vi "Inverter_write_read_json text step array.vi"(8 "error in":errorcluster, 9 "json_array_from_file":T1[](array[typedef])=[{"step_description (prompt)"="(prompt)", "save results"=FALSE, "step_type"=enum."prompt", "Step_name"="", "bool"=[], "data_unit"=enum."bool", "dbl"=[], "I32"=[], "string"=[]}, {"step_description (prompt)"="set hipot Voltage", "save results"=FALSE, "step_type"=enum."wait (sec)", "Step_name"="", "bool"=[], "data_unit"=enum."DBL", "dbl"=[], "I32"=[], "string"=[]}, {"step_description (prompt)"="read hipot v", "save results"=FALSE, "step_type"=enum."default", "Step_name"="", "bool"=[], "data_unit"=enum."bool", "dbl"=[], "I32"=[], "string"=[]}] {"dbl" format="%.3f"}, 10 "write_read":T4=enum."read", 11 "File Path":path) -> (0 "error out":errorcluster, 1 "steps array out":T1[](array[typedef]) {"dbl" format="%.3f"}, 3 "File Path":path)   [LabVIEW 2020]
uses:
  controls/Inverter_step.ctl
  controls/Inverter_step_type.ctl
  MPB/controls/data type.ctl
  MPB/controls/write_read.ctl
  3e47bdee-b09f-426d-96e8-78c270cf6aec.vi
  <vilib>/JDP Science/JSONtext/JSON text to Variant.vi
  <vilib>/JDP Science/JSONtext/JSONtext.lvlib
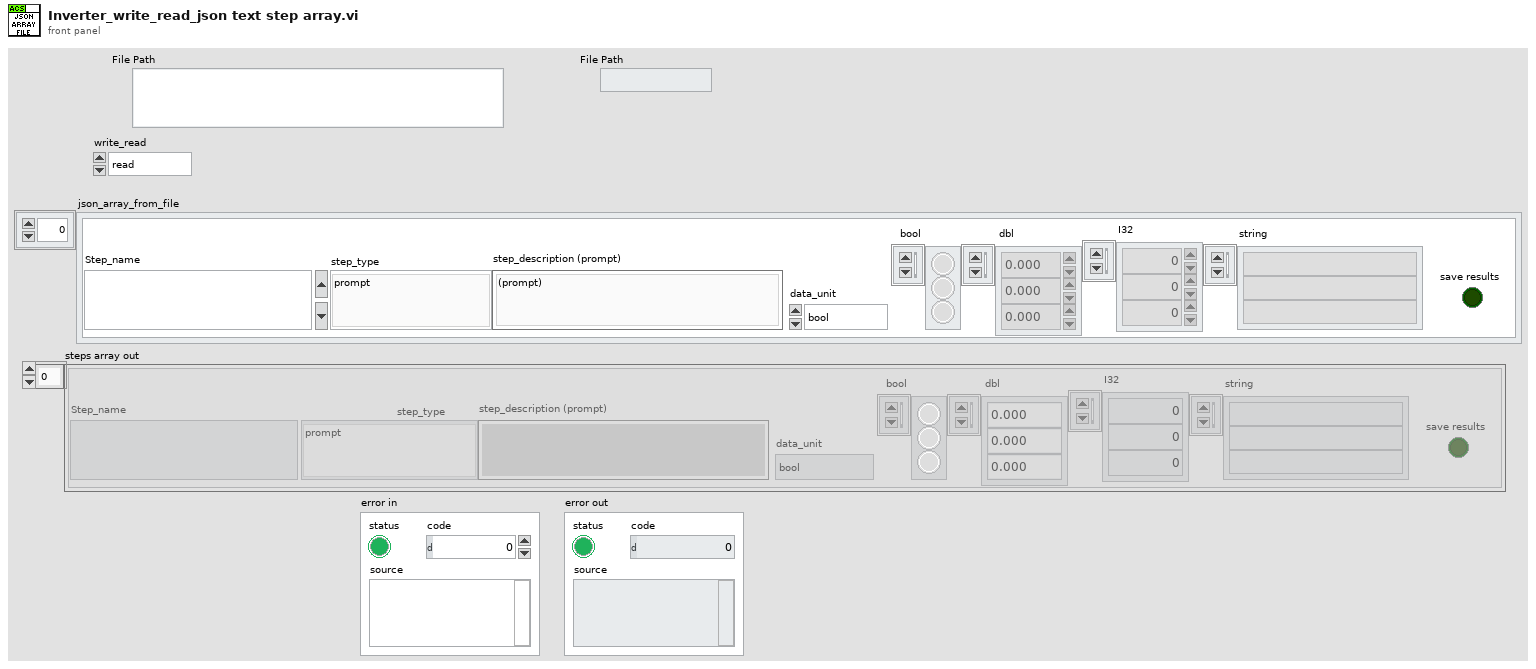
[diagram p1: front panel]
types:
  T1 = typedef "Inverter_step.ctl" = cluster{"step_description (prompt)":string, "save results":bool, "step_type":T2, "Step_name":string, "bool":bool[], "data_unit":T3, "dbl":dbl[], "I32":i32[], "string":string[]}
  T2 = typedef "Inverter_step_type.ctl" = enum16{"default", "prompt", "init_12V_power_supply", "12V_power supply on_off", "write_PLC", "read_PLC", "DAQ_Read", "DAQ_Write", "run .bat file", "display_version", "set flow rate", "init_chroma", "set_chroma_V", "set_chroma_ramp", "wait (sec)", "end_of_test", "record_pass_fail"}
  T3 = typedef "data type.ctl" = enum16{"bool", "string", "I32", "DBL"}
  T4 = typedef "write_read.ctl" = enum16{"write", "read"}
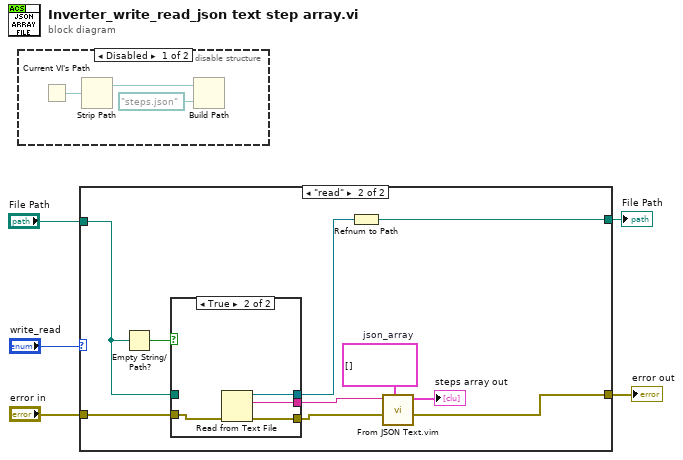
[diagram p0: block diagram]
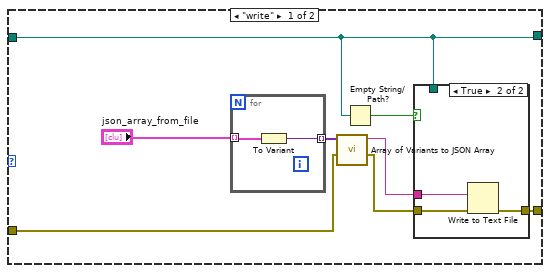
[diagram p3: hidden frame]
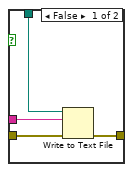
[diagram p4: hidden frame]
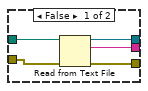
[diagram p5: hidden frame]
diagram:
  n1 = disable-structure shown="Disabled" {
    frame Disabled {
      n2 = Current VI's Path() -> (path=w8:path)
      n3 = Strip Path(path=w8) -> (stripped path=w7:path)  [unwired: 1 out]
      n4 = Build Path(base path=w7, name or relative path=path "steps.json") -> ()  [unwired: 1 out]
    }
    frame Enabled {
    }
  }
  n5 = case shown="\"read\"" "write_read" {
    tunnel: "error in" -> [w13 w31]
    tunnel: [w11 w33] -> w3
    tunnel: [w9 w32] -> w2
    tunnel: "File Path" -> [w9 w29]
    frame "write" {
      n6 = for {
        tunnel: "json_array_from_file" -> [w24] mode=indexing
        tunnel: [w25] -> w16 mode=indexing
        n7 = To Variant(anything=w24) -> (Variant=w25:variant)
      }
      n8 = call <vilib>:"Array of Variants to JSON Array.vi"("error in (no error)"=w13, "Array of Variants"=w16) -> ("error out"=w12:errorcluster, "<JSON>"=w15:string)  [unwired: 8 in]
      n9 = Empty String/Path?(string/path=w9) -> (empty?=w10:bool)
      n10 = case shown="True" w10 {
        tunnel: w15 -> [w20 w23]
        tunnel: w12 -> [w19 w22]
        tunnel: [w18 w21] -> w11
        tunnel: w9 -> [w17 _]
        frame False {
          n11 = Write to Text File(file (use dialog)=w17, text=w20, error in=w19) -> (error out=w18:errorcluster)  [unwired: 1 in, 2 out]
        }
        frame True {
          n12 = Write to Text File(text=w23, error in=w22) -> (error out=w21:errorcluster)  [unwired: 2 in, 2 out]
        }
      }
    }
    frame "read" {
      w34 = T1[] []  # json_array
      n13 = Empty String/Path?(string/path=w29) -> (empty?=w30:bool)
      n14 = case shown="True" w30 {
        tunnel: w31 -> [w37 w42]
        tunnel: w29 -> [w40 _]
        tunnel: [w39 w44] -> w28
        tunnel: [w38 w43] -> w27
        tunnel: [w36 w41] -> w26
        frame False {
          n15 = Read from Text File(file (use dialog)=w40, error in=w37) -> (refnum out=w39:refnum<file>, text=w38:string, error out=w36:errorcluster)  [unwired: 2 in, 1 out]
        }
        frame True {
          n16 = Read from Text File(error in=w42) -> (refnum out=w44:refnum<file>, text=w43:string, error out=w41:errorcluster)  [unwired: 3 in, 1 out]
        }
      }
      n17 = Refnum to Path(1:w28) -> (0:w32:path)
      n18 = call "From JSON Text.vim"("Data Type and Default Value"=w34, "error in (no error)"=w26, "JSON"=w27) -> ("error out"=w33:errorcluster, "Data out"=→"steps array out":T1[])  [unwired: 7 in]
    }
  }
  "error out" <- w3
  "File Path" <- w2
